vi "Cluster Item section.vi"(8 "error in (no error)":errorcluster, 10 "indent":i32, 11 "count":i32) -> (0 "error out":errorcluster, 3 "Cluster Item":T1)   [LabVIEW 2020, in "DSF Configuration Utility.lvlib"]
uses:
  DSF Configuration Utility.lvlib
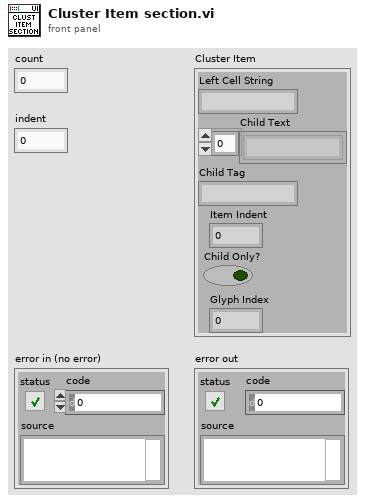
[diagram p1: front panel]
types:
  T1 = cluster{"Left Cell String":string, "Child Text":string[], "Child Tag":string, "Item Indent":i32, "Child Only?":bool, "Glyph Index":i32}
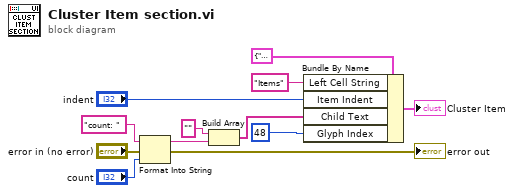
[diagram p0: block diagram]
diagram:
  n1 = Format Into String(initial string="count: ", error in="error in (no error)", "count") -> (resulting string=w3:string, error out=→"error out":errorcluster)  [unwired: 1 in]
  n2 = Build Array("" ("element"), w3) -> (w9:string[])
  n3 = Bundle By Name(cluster=T1 {"Left Cell String"="", "Child Text"=[], "Child Tag"="", "Item Indent"=0, "Child Only?"=FALSE, "Glyph Index"=0} ("Item"), "Left Cell String"="Items", "Item Indent"="indent", "Child Text"=w9, "Glyph Index"=48) -> (→"Cluster Item":T1)
